vi "niRFUtil RFHS Channelizer ChannelizerArrayCommon_CSG.vi"(0 "Channelizer Ref":refnum<data-value>, 1 "Reset":bool, 2 "Reset Cnt":i64=-1, 3 "Caller Flags":T1 items=["None"=0, "Skip Stage 1"=1, "FFT Stage"=2, "Frequency Shift"=4, "Finite Buffer"=8, "Reset"=16, "Input Len Estimate"=32, "C buffers"=64, "Input From Ref"=128, "Use Pretrigger Data"=256], 5 "Data":csg[](array[numeric]), 7 "Data Subset":T2={"Offset"=0, "Length"=-1}, 11 "error in (no error)":errorcluster, 13 "CPU Context":string) -> (4 "Channelizer Ref (out)":refnum<data-value>, 6 "Channel Data":csg[](array[numeric]), 8 "Data (out)":csg[](array[numeric]), 10 "Time":u32, 14 "Channel Data Len":u32[](array[numeric]), 15 "error out":errorcluster)   [LabVIEW 2015, in "niRFUtil.lvlib"]
uses:
  niRFUtil.lvlib
  Utilities/niRFUtil RFHS Util Data Subset.ctl
  Includes/niRFUtil RFHS Channelizer ChannelizerInfo CSG.ctl
  Includes/niRFUtil RFHS Channelizer FilterRef.ctl
  Includes/niRFUtil RFHS Channelizer ChannelizerBufferingMode.ctl
  Utilities/Data FIFO/niRFUtil RFHS FIFO Reference.ctl
  Utilities/Data FIFO/niRFUtil RFHS FIFO.ctl
  Includes/niRFUtil RFHS Channelizer ChannelizerType.ctl
  Includes/niRFUtil RFHS Channelizer ChannelizerFlags.ctl
panel:
  out "tmpBuf 2":csg[](array[numeric])
  out "tmpBuf":csg[](array[numeric])
  out "Filtered Data 2":csg[](array[numeric])
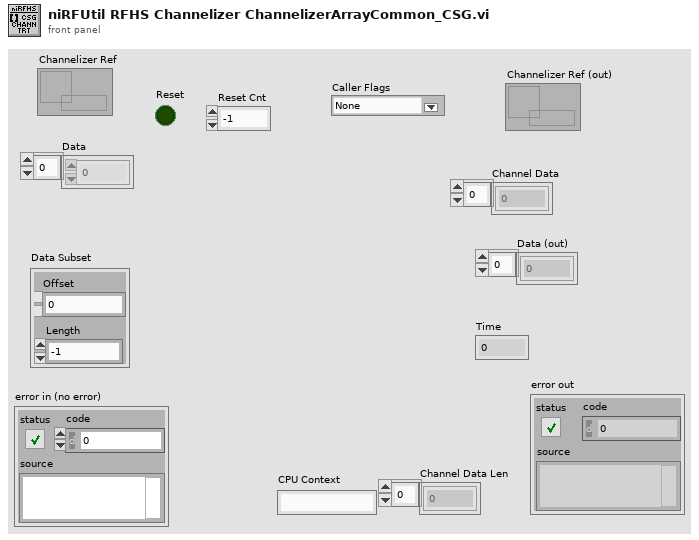
[diagram p1: front panel]
types:
  T1 = typedef "niRFUtil.lvlib/niRFUtil RFHS Channelizer ChannelizerFlags.ctl" = u32
  T2 = typedef "niRFUtil.lvlib/niRFUtil RFHS Util Data Subset.ctl" = cluster{"Offset":i32, "Length":i32}
  T3 = typedef "niRFUtil.lvlib/niRFUtil RFHS Channelizer ChannelizerType.ctl" = enum32{"Auto", "Frequency Shift Only", "Resampler Only"}
  T4 = typedef "niRFUtil.lvlib/niRFUtil RFHS Channelizer ChannelizerInfo CSG.ctl" = cluster{"Filter LVRef":T5, "Mode":T6, "History":csg[], "Buffer":csg[], "FIFO":T7, "History Len":u32, "Float Cache":csg[], "Double Cache":cdb[], "Type":T3, "Resample Phase":dbl, "fft1Descriptors":u64[], "fft2Descriptors":u64[], "FFT tBuf":csg[], "guardBandLen":i32, "FFT History":csg[], "FFT History Len":u32, "FFTInitDone":u32, "FFT Filter LVRefs":T5[], "FFT fc Offs":u32[], "fft2Sizes":u32[], "BufferW":u32[], "BufferR":u32[], "Buff Off":u32[], "Phase0 (fshift)":dbl[], "Phase (fshift)":dbl[], "fs phase step":dbl[], "Resample Step":dbl, "Flags":T1, "Reset Cnt":i64, "Filter Pass":u32, "Stages":variant[]}
  T5 = typedef "niRFUtil.lvlib/niRFUtil RFHS Channelizer FilterRef.ctl" = cluster{"Ref":u64, "GUID":u64, "Upsample":i32, "Downsample":i32, "Size":i32, "Num Taps":i32}
  T6 = typedef "niRFUtil.lvlib/niRFUtil RFHS Channelizer ChannelizerBufferingMode.ctl" = enum32{"Unbuffered", "Finite", "Continuous"}
  T7 = typedef "niRFUtil.lvlib/niRFUtil RFHS FIFO Reference.ctl" = cluster{"Read Lock":refnum<data-value>, "Info":T8, "Write Lock":refnum<data-value>}
  T8 = typedef "niRFUtil.lvlib/niRFUtil RFHS FIFO.ctl" = cluster{"ID":u64, "Length":u32}
  T9 = typedef "niRFUtil.lvlib/niRFUtil RFHS Channelizer CPUInfo.ctl" = cluster{"Num CPUs":u32, "Points/CPU":u32, "CPU Context":T10, "Mode":i32}
  T10 = typedef "niRFUtil.lvlib/niRFUtil RFHS Util CPU Context.ctl" = u64[]
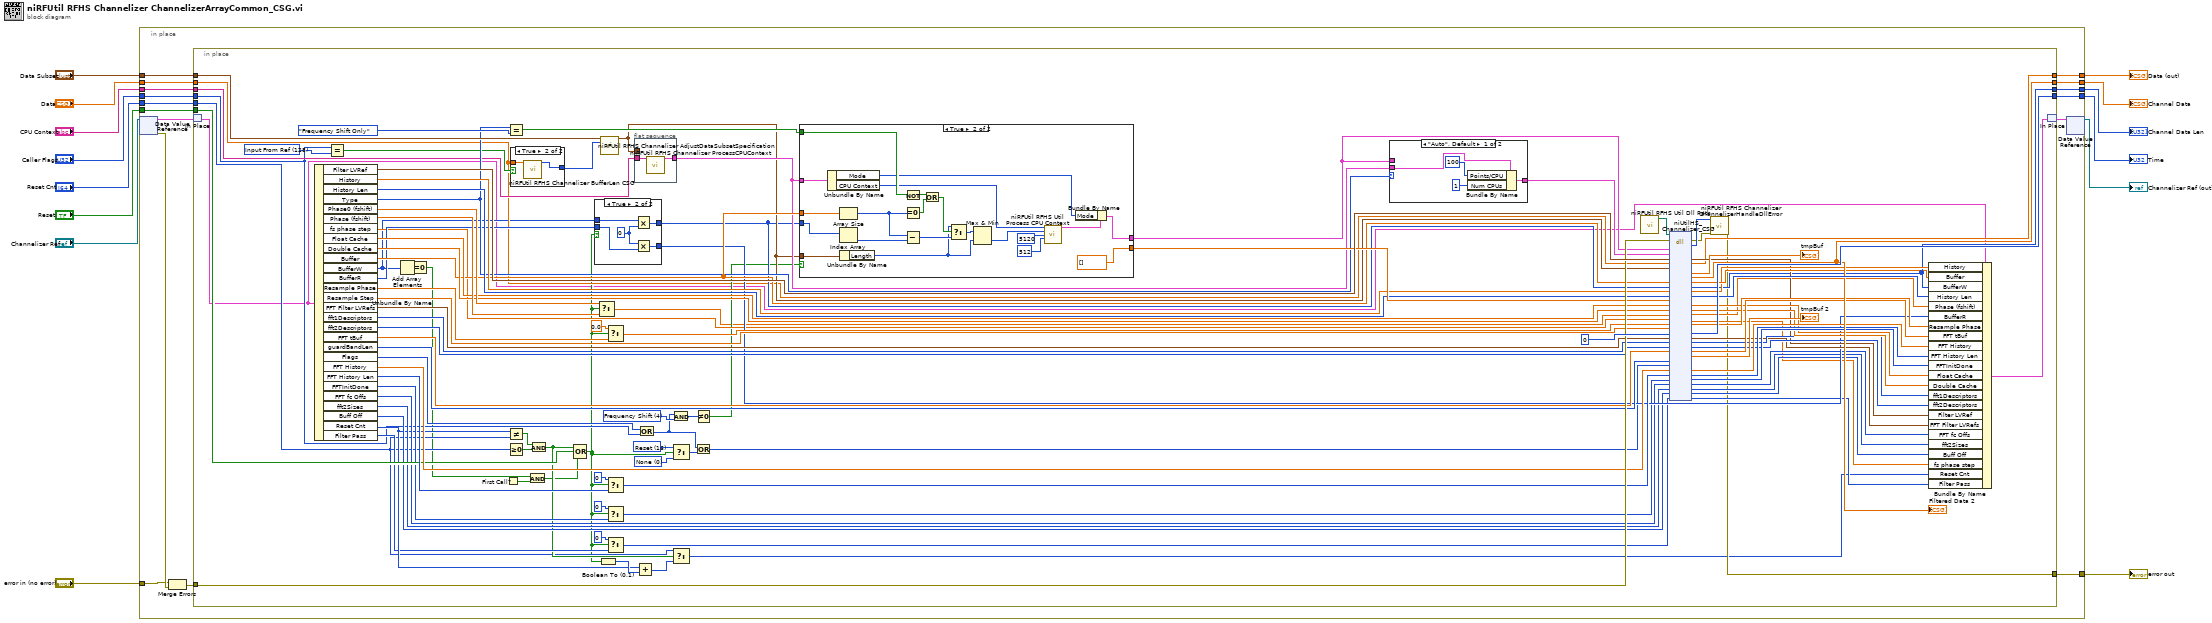
[diagram p0: block diagram]
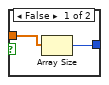
[diagram p2: hidden frame]
diagram:
  n1 = in-place {
    in-place-border: "error in (no error)" -> [w17]
    in-place-border: "Data" -> [w26]
    in-place-border: "Reset" -> [w24]
    in-place-border: [w30] -> w2
    in-place-border: [w27] -> w12
    in-place-border: [w29] -> w11
    in-place-border: "CPU Context" -> [w25]
    in-place-border: "Data Subset" -> [w28]
    in-place-border: [w21] -> w5
    in-place-border: "Reset Cnt" -> [w20]
    in-place-border: [w19] -> w3
    in-place-border: "Caller Flags" -> [w15]
    n2 = in-place-dvr #1 ("Data Value Reference Read / Write Element")("Channelizer Ref") -> (w22:T4, w18:errorcluster)
    n3 = Merge Errors(w17, w18) -> (w16:errorcluster)
    n4 = in-place {
      in-place-border: [w49] -> w30
      in-place-border: [w138] -> w29
      in-place-border: w28 -> [w137]
      in-place-border: [w134] -> w27
      in-place-border: w16 -> [w132]
      in-place-border: w26 -> [w39]
      in-place-border: w25 -> [w115]
      in-place-border: w24 -> [w95]
      in-place-border: [w71] -> w21
      in-place-border: w20 -> [w47]
      in-place-border: [w61] -> w19
      in-place-border: w15 -> [w42]
      w41 = T1 128 items=["None"=0, "Skip Stage 1"=1, "FFT Stage"=2, "Frequency Shift"=4, "Finite Buffer"=8, "Reset"=16, "Input Len Estimate"=32, "C buffers"=64, "Input From Ref"=128] ("y")
      w54 = T1 16 items=["None"=0, "Skip Stage 1"=1, "FFT Stage"=2, "Frequency Shift"=4, "Finite Buffer"=8, "Reset"=16, "Input Len Estimate"=32] ("Flags")
      w55 = T1 0 items=["None"=0, "Skip Stage 1"=1, "FFT Stage"=2, "Frequency Shift"=4, "Finite Buffer"=8] ("Flags")
      w70 = T1 4 items=["None"=0, "Skip Stage 1"=1, "FFT Stage"=2, "Frequency Shift"=4] ("y")
      n5 = in-place-match #2(w22) -> (w31:T4)
      n6 = Unbundle By Name(w31) -> ("Filter LVRef"=w135:T5, "History"=w127:csg[], "History Len"=w126:u32, "Type"=w125:T3, "Phase0 (fshift)"=w124:dbl[], "Phase (fshift)"=w123:dbl[], "fs phase step"=w72:dbl[], "Float Cache"=w122:csg[], "Double Cache"=w121:cdb[], "Buffer"=w117:csg[], "BufferW"=w37:u32[], "BufferR"=w83:u32[], "Resample Phase"=w111:dbl, "Resample Step"=w112:dbl, "FFT Filter LVRefs"=w108:T5[], "fft1Descriptors"=w107:u64[], "fft2Descriptors"=w106:u64[], "FFT tBuf"=w105:csg[], "guardBandLen"=w104:i32, "Flags"=w44:T1, "FFT History"=w101:csg[], "FFT History Len"=w97:u32, "FFTInitDone"=w94:u32, "FFT fc Offs"=w77:u32[], "fft2Sizes"=w76:u32[], "Buff Off"=w75:u32[], "Reset Cnt"=w64:i64, "Filter Pass"=w59:u32)
      n7 = Equal?(x=w42, y=w41) -> (x = y?=w40:bool)
      n8 = Add Array Elements(numeric array=w37) -> (sum=w35:u32)
      n9 = Equal To 0?(x=w35) -> (x = 0?=w34:bool)
      n10 = First Call?() -> (First Call?: T/F=w36:bool)
      n11 = Equal?(x=w125, y=niRFUtil_RFHS_Channelizer_ChannelizerType."Frequency Shift Only") -> (x = y?=w116:bool)
      n12 = Not Equal?(x=w64, y=w47) -> (x != y?=w63:bool)
      n13 = Greater Or Equal To 0?(x=w47) -> (x >= 0?=w62:bool)
      n14 = case shown="True" w40 {
        tunnel: w39 -> [w140 w142]
        tunnel: [w139 w141] -> w38
        frame False {
          n15 = Array Size(array=w140) -> (size(s)=w139:i32)
        }
        frame True {
          n16 = call "niRFUtil RFHS Channelizer BufferLen CSG.vi"("Buffer"=w142) -> ("Length"=w141:i32)  [unwired: 14 in]
        }
      }
      n17 = And(x=w34, y=w36) -> (x .and. y?=w33:bool)
      n18 = And(x=w63, y=w62) -> (x .and. y?=w48:bool)
      n19 = Compound Arithmetic op=OR(w48, w95, w33) -> (w32:bool)
      n20 = case shown="True" w32 {
        tunnel: w37 -> [w144 w149]
        tunnel: [w144 w148] -> w81
        tunnel: [w143 w145] -> w82
        tunnel: w83 -> [w143 w146]
        frame False {
        }
        frame True {
          w147 = u32 0 ("t")
          n21 = Multiply(x=w149, y=w147) -> (x*y=w148:u32[])
          n22 = Multiply(x=w147, y=w146) -> (x*y=w145:u32[])
        }
      }
      n23 = Select(t=w124, s=w32, f=w123) -> (s? t:f=w67:dbl[])
      n24 = Boolean To (0,1)(Boolean=w32) -> (0, 1=w65:i16)
      n25 = call "niRFUtil RFHS Channelizer AdjustDataSubsetSpecification.vi"("Data Subset"=w137, "Max Length"=w38) -> ("Data Subset (adjusted)"=w85:T2)  [unwired: 13 in]
      n26 = Select(t=0.0, s=w32, f=w111) -> (s? t:f=w109:dbl)
      n27 = Select(t=u32 0, s=w32, f=w97) -> (s? t:f=w96:u32)
      n28 = Select(t=u32 0, s=w32, f=w94) -> (s? t:f=w60:u32)
      n29 = Select(t=u32 0, s=w32, f=w59) -> (s? t:f=w57:u32)
      n30 = flat-sequence {
        tunnel: w115 -> [w151]
        tunnel: [w150] -> w114
        tunnel: w85 -> [_]
        frame #0 {
          n31 = call "niRFUtil RFHS Channelizer ProcessCPUContext.vi"("CPU Context"=w151) -> ("Exec Config"=w150:T9)  [unwired: 14 in]
        }
      }
      n32 = Add(x=w64, y=w65) -> (x+y=w46:i64)
      n33 = Or(x=w44, y=w42) -> (x .or. y?=w43:T1)
      n34 = And(x=w43, y=w70) -> (x .and. y?=w69:T1)
      n35 = Select(t=w54, s=w32, f=w55) -> (s? t:f=w53:T1)
      n36 = Select(t=w47, s=w48, f=w46) -> (s? t:f=w45:i64)
      n37 = Not Equal To 0?(x=w69) -> (x != 0?=w68:bool)
      n38 = Or(x=w43, y=w53) -> (x .or. y?=w52:T1)
      n39 = case shown="True" w68 {
        tunnel: w85 -> [_ w175]
        tunnel: w114 -> [_ w164]
        tunnel: [_ dbl[] [] ("double precision float")] -> w130
        tunnel: [_ w165] -> w74
        tunnel: w117 -> [_ w174]
        tunnel: w81 -> [_ w161]
        tunnel: w116 -> [_ w167]
        frame False {
        }
        frame True {
          n40 = Unbundle By Name(w164) -> ("Mode"=w163:i32, "CPU Context"=w162:T10)
          n41 = Array Size(array=w174) -> (size(s)=w173:i32)
          n42 = Index Array(array=w161) -> (element=w160:u32)  [unwired: 1 in]
          n43 = Unbundle By Name(w175) -> ("Length"=w158:i32)
          n44 = Not(x=w167) -> (.not. x?=w168:bool)
          n45 = Equal To 0?(x=w173) -> (x = 0?=w172:bool)
          n46 = Subtract(x=w173, y=w160) -> (x-y=w171:u32)
          n47 = Or(x=w168, y=w172) -> (x .or. y?=w169:bool)
          n48 = Select(t=w158, s=w169, f=w171) -> (s? t:f=w157:u32)
          n49 = Max & Min(x=w157, y=w158) -> (min(x,y)=w170:u32)  [unwired: 1 out]
          n50 = call "niRFUtil RFHS Util Process CPU Context.vi"("CPU Context"=w162, "Points"=w170, "Threshold"=5120, "Multiple"=512) -> ("Exec Config"=w166:T9)  [unwired: 10 in, 1 out]
          n51 = Bundle By Name(cluster=w166, "Mode"=w163) -> (w165:T9)
        }
      }
      n52 = case shown="\"Auto\", Default" w125 {
        tunnel: [w153 _] -> w128
        tunnel: w114 -> [w152 _]
        tunnel: w74 -> [_ _]
        frame "Auto", Default {
          n53 = Bundle By Name(cluster=w152, "Points/CPU"=u32 100, "Num CPUs"=u32 1) -> (w153:T9)
        }
        frame "Frequency Shift Only" {
        }
      }
      n54 = call "niRFUtil RFHS Util Dll Path.vi"() -> ("Path"=w84:path)  [unwired: 7 in, 4 out]
      n55 = dll-call lib="?" fn="niUtilHS_Channelizer_CSG"(path in=w84, error in=w132, "ecFrequencyShift"=w74, "ecResampler"=w128, "filterRef"=w135, "iBuf"=w39, "dataSubset"=w85, "internalOBuf"=w117, "bufW"=w81, "historyBuf"=w127, "historyLen"=w126, "startState"=w130, "floatCache"=w122, "doubleCache"=w121, "fsPhase"=w67, "fsPhaseStep"=w72, "resample phase"=w109, "resample phaseStep"=w112, "time"=u32 0, "FFTFilterRefs"=w108, "fft1Descriptors"=w107, "fft2Descriptors"=w106, "FFTTempBuf"=w105, "guardBandLen"=w104, "flags"=w52, "FFTHistory"=w101, "FFTHistoryLen"=w96, "FFTInitDone"=w60, "FFT fc Offs"=w77, "fft2Sizes"=w76, "BufOff"=w75, "filterPass"=w57) -> (error out=w50:errorcluster, "return type"=w51:i32, "filterRef"=w87:T5, "iBuf"=w71:csg[], "tmpBuf"=→"tmpBuf":csg[], "Filtered Data 2"=w134:csg[], "internalOBuf"=w120:csg[], "bufW"=w61:u32[], "historyBuf"=w118:csg[], "historyLen"=w136:u32, "floatCache"=w91:csg[], "doubleCache"=w90:cdb[], "fsPhase"=w66:dbl[], "fsPhaseStep"=w73:dbl[], "resample phase"=w113:dbl, "time"=w138:u32, "FFTFilterRefs"=w86:T5[], "fft1Descriptors"=w89:u64[], "fft2Descriptors"=w88:u64[], "FFTTempBuf"=w102:csg[], "tmpBuf 2"=→"tmpBuf 2":csg[], "FFTHistory"=w100:csg[], "FFTHistoryLen"=w99:i32, "FFTInitDone"=w92:u32, "FFT fc Offs"=w80:u32[], "fft2Sizes"=w79:u32[], "BufOff"=w78:u32[], "filterPass"=w56:u32)  [unwired: 11 in, 1 out]
      "Filtered Data 2" <- w134
      n56 = call "niRFUtil RFHS Channelizer ChannelizerHandleDllError.vi"("Error"=w51, "error in (no error)"=w50) -> ("error out"=w49:errorcluster)  [unwired: 13 in]
      n57 = Bundle By Name(cluster=w31, "History"=w118, "Buffer"=w120, "BufferW"=w61, "History Len"=w136, "Phase (fshift)"=w66, "BufferR"=w82, "Resample Phase"=w113, "FFT tBuf"=w102, "FFT History"=w100, "FFT History Len"=w99, "FFTInitDone"=w92, "Float Cache"=w91, "Double Cache"=w90, "fft1Descriptors"=w89, "fft2Descriptors"=w88, "Filter LVRef"=w87, "FFT Filter LVRefs"=w86, "FFT fc Offs"=w80, "fft2Sizes"=w79, "Buff Off"=w78, "fs phase step"=w73, "Reset Cnt"=w45, "Filter Pass"=w56) -> (w119:T4)
      n58 = in-place-match #2(w119) -> (w23:T4)
    }
    n59 = in-place-dvr #1(w23) -> (→"Channelizer Ref (out)":refnum<data-value>)  [unwired: 1 out]
  }
  "error out" <- w2
  "Channel Data" <- w12
  "Time" <- w11
  "Data (out)" <- w5
  "Channel Data Len" <- w3
